vi "splitIntoCommandElementPairs.vi"(8 "error in (no error)":errorcluster, 10 "command":string, 11 "CommandProcessor in":refnum<class "CommandProcessor.lvclass">) -> (0 "error out":errorcluster, 3 "CommandProcessor out":refnum<class "CommandProcessor.lvclass">)   [LabVIEW 2011, in "Tools.lvlib" / "Interpreters.lvlib" / "CommandProcessor.lvclass"]
uses:
  CommandProcessor.lvclass
  CommandProcessor.lvclass/CommandProcessor.ctl
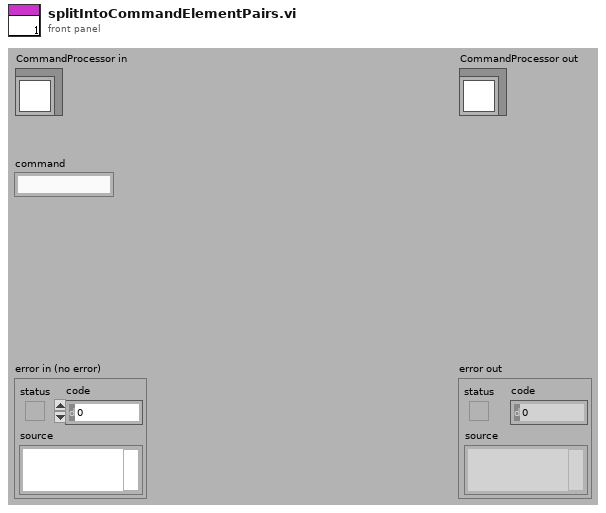
[diagram p1: front panel]
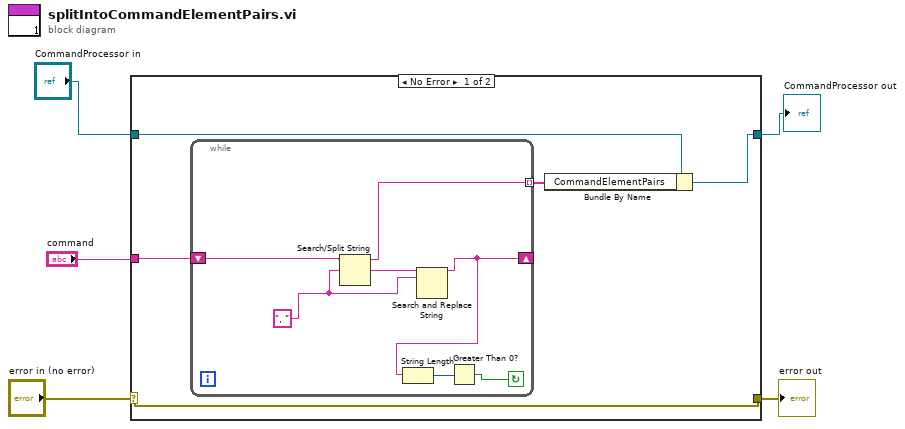
[diagram p0: block diagram]
diagram:
  n1 = case shown="No Error" "error in (no error)" {
    selector: "error in (no error)" -> [w10 w19]
    tunnel: [w10 w19] -> w4
    tunnel: [w6 w18] -> w2
    tunnel: "CommandProcessor in" -> [w8 w18]
    tunnel: "command" -> [w9 _]
    frame No Error {
      n2 = while {
        shift-right: [w12] -> _
        shift-left: w9 -> [w13]
        tunnel: [w15] -> w7 mode=indexing
        stop <- w16 continue-if-true
        w11 = ", "
        n3 = Search/Split String(string=w13, search string/char (-)=w11) -> (substring before match=w15:string, match + rest of string=w14:string)  [unwired: 1 in, 1 out]
        n4 = Search and Replace String(input string=w14, search string=w11) -> (result string=w12:string)  [unwired: 6 in, 3 out]
        n5 = String Length(string=w12) -> (length=w17:i32)
        n6 = Greater Than 0?(x=w17) -> (x > 0?=w16:bool)
      }
      n7 = Bundle By Name(cluster=w8, "CommandElementPairs"=w7) -> (w6:refnum<class "CommandProcessor.lvclass">)
    }
    frame Error {
    }
  }
  "error out" <- w4
  "CommandProcessor out" <- w2
